vi "Approx Equal (1D).vi"(4 "Y":dbl[](array[numeric]), 5 "X":dbl[](array[numeric])) -> (1 "X approx Y?":bool)   [LabVIEW 2020]
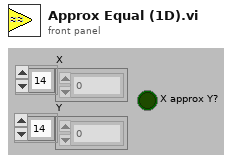
[diagram p1: front panel]
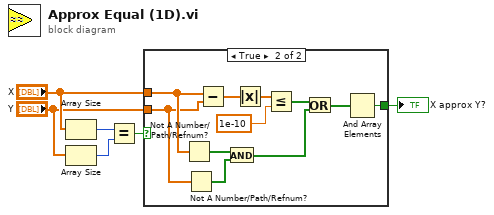
[diagram p0: block diagram]
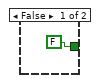
[diagram p2: hidden frame]
diagram:
  n1 = Array Size(array="X") -> (size(s)=w3:i32)
  n2 = Array Size(array="Y") -> (size(s)=w2:i32)
  n3 = Equal?(x=w3, y=w2) -> (x = y?=w1:bool)
  n4 = case shown="True" w1 {
    tunnel: "X" -> [_ w15]
    tunnel: "Y" -> [_ w14]
    tunnel: [FALSE w16] -> w6
    frame False {
    }
    frame True {
      n5 = Not A Number/Path/Refnum?(number/path/refnum=w15) -> (NaN/Path/Refnum?=w13:bool[])
      n6 = Not A Number/Path/Refnum?(number/path/refnum=w14) -> (NaN/Path/Refnum?=w12:bool[])
      n7 = Subtract(x=w15, y=w14) -> (x-y=w18:dbl[])
      n8 = And(x=w13, y=w12) -> (x .and. y?=w10:bool[])
      n9 = Absolute Value(x=w18) -> (abs(x)=w17:dbl[])
      n10 = Less Or Equal?(x=w17, y=1e-10) -> (x <= y?=w11:bool[])
      n11 = Or(x=w11, y=w10) -> (x .or. y?=w9:bool[])
      n12 = And Array Elements(Boolean array=w9) -> (logical AND=w16:bool)
    }
  }
  "X approx Y?" <- w6
